vi "AlliGator Check Phasor Plot Destination.vi"(9 "Second Plot Name":string, 10 "First Plot Name":string, 11 "Phasor Plot Destination in":T1) -> (1 "Destination Plot Name":string, 3 "Phasor Plot Destination out":T1)   [LabVIEW 2021, in "AlliGator Phasor Graph.lvlib"]
doc: "Checks whether a Phasor Plot Destination is valid (i.e. a valid plot was provided: non empty name) as a destination.\n\nIf not a valid destination, the new plot will be appended to the graph."
uses:
  AlliGator Phasor Graph.lvlib
  AlliGator Phasor Plot Destination.ctl
panel:
  # "see the AlliGator License on the block diagram (Ctrl+E or Window:Show Block Diagram)"
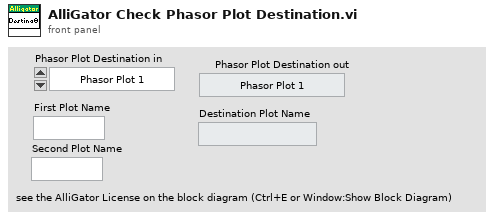
[diagram p1: front panel]
types:
  T1 = typedef "AlliGator Phasor Graph.lvlib/AlliGator Phasor Plot Destination.ctl" = enum32{"Phasor Plot 1", "Phasor Plot 2", "New Phasor Plot"}
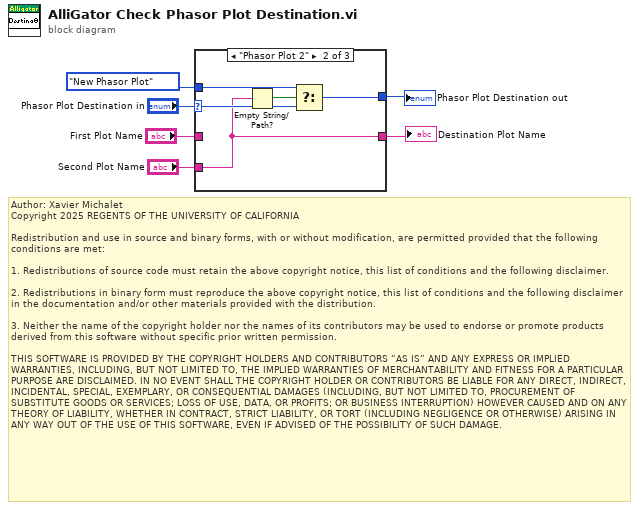
[diagram p0: block diagram]
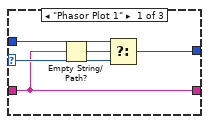
[diagram p2: hidden frame]
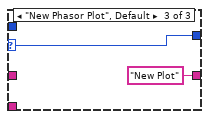
[diagram p3: hidden frame]
diagram:
  # "Author: Xavier Michalet\nCopyright 2025 REGENTS OF THE UNIVERSITY OF CALIFORNIA\n\nRedistribution and use in source and binary forms, with or without modification, are permitted provided that the following conditions are met:\n\n1. Redistributions of source code must retain the above copyright notice, this list of conditions and the following disclaimer.\n\n2. Redistributions in binary form must reproduce the above copyright notice, this list of conditions and the following disclaimer in the documentation and/or other materials provided with the distribution.\n\n3. Neither the name of the copyright holder nor the names of its contributors may be used to endorse or promote products derived from this software without specific prior written permission.\n\nTHIS SOFTWARE IS PROVIDED BY THE COPYRIGHT HOLDERS AND CONTRIBUTORS “AS IS” AND ANY EXPRESS OR IMPLIED WARRANTIES, INCLUDING, BUT NOT LIMITED TO, THE IMPLIED WARRANTIES OF MERCHANTABILITY AND FITNESS FOR A PARTICULAR PURPOSE ARE DISCLAIMED. IN NO EVENT SHALL THE COPYRIGHT HOLDER OR CONTRIBUTORS BE LIABLE FOR ANY DIRECT, INDIRECT, INCIDENTAL, SPECIAL, EXEMPLARY, OR CONSEQUENTIAL DAMAGES (INCLUDING, BUT NOT LIMITED TO, PROCUREMENT OF SUBSTITUTE GOODS OR SERVICES; LOSS OF USE, DATA, OR PROFITS; OR BUSINESS INTERRUPTION) HOWEVER CAUSED AND ON ANY THEORY OF LIABILITY, WHETHER IN CONTRACT, STRICT LIABILITY, OR TORT (INCLUDING NEGLIGENCE OR OTHERWISE) ARISING IN ANY WAY OUT OF THE USE OF THIS SOFTWARE, EVEN IF ADVISED OF THE POSSIBILITY OF SUCH DAMAGE."
  n1 = case shown="\"Phasor Plot 2\"" "Phasor Plot Destination in" {
    selector: "Phasor Plot Destination in" -> [w10 w15 w18]
    tunnel: "First Plot Name" -> [w7 _ _]
    tunnel: AlliGator_Phasor_Plot_Destination."New Phasor Plot" ("Phasor Plot Destination in") -> [w9 w14 _]
    tunnel: [w8 w13 w18] -> w4
    tunnel: "Second Plot Name" -> [_ w12 _]
    tunnel: [w7 w12 "New Plot" ("Second Plot Name")] -> w2
    frame "Phasor Plot 1" {
      n2 = Empty String/Path?(string/path=w7) -> (empty?=w11:bool)
      n3 = Select(t=w9, s=w11, f=w10) -> (s? t:f=w8:T1)
    }
    frame "Phasor Plot 2" {
      n4 = Empty String/Path?(string/path=w12) -> (empty?=w16:bool)
      n5 = Select(t=w14, s=w16, f=w15) -> (s? t:f=w13:T1)
    }
    frame "New Phasor Plot", Default {
    }
  }
  "Phasor Plot Destination out" <- w4
  "Destination Plot Name" <- w2
